vi "LibXML_ReadXMLTreeSerial.vi"(8 "error in":errorcluster, 9 "parent":u32, 10 "XML-tree in":T1[](array[typedef]), 11 "start node":u32) -> (0 "error out":errorcluster, 2 "XML-tree out":T1[](array[typedef]), 3 "copy of start node":u32)   [LabVIEW 2019, in "Tools.lvlib" / "LibXML.lvlib"]
uses:
  LibXML.lvlib
  LibXML_Element.ctl
  LibXML_Attribute.ctl
  LibXML_NavigateDirection.ctl
  LibXML_GetNodeStrPtr.vi
  LibXML_GetNodeResolvedContentStrPointer.vi
  LibXML_GetStringLength.vi
  LibXML_CopyString.vi
  Error Cluster From Error Code_subroutine.vi
  <vilib>/Utility/error.llb/Trim Whitespace.vi
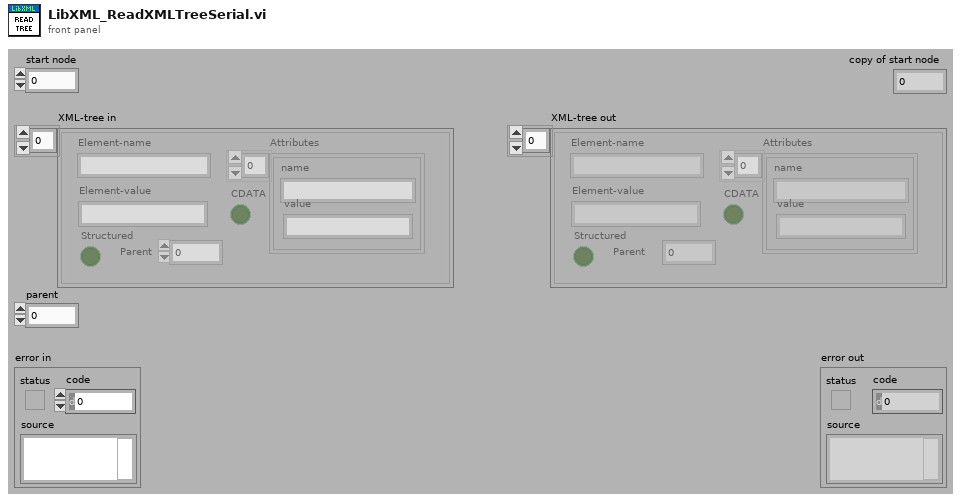
[diagram p1: front panel]
types:
  T1 = typedef "Tools.lvlib/LibXML.lvlib/LibXML_Element.ctl" = cluster{"Element-name":string, "Attributes":T2[], "Element-value":string, "CDATA":bool, "Parent":i32, "Structured":bool}
  T2 = typedef "Tools.lvlib/LibXML.lvlib/LibXML_Attribute.ctl" = cluster{"name":string, "value":string}
  T3 = typedef "Tools.lvlib/LibXML.lvlib/LibXML_NavigateDirection.ctl" = enum16{"NOP", "first child", "last child", "parent", "next", "prev"}
  T4 = enum16{"nothing", "element", "attribute", "text", "cdata", "5 or more"}
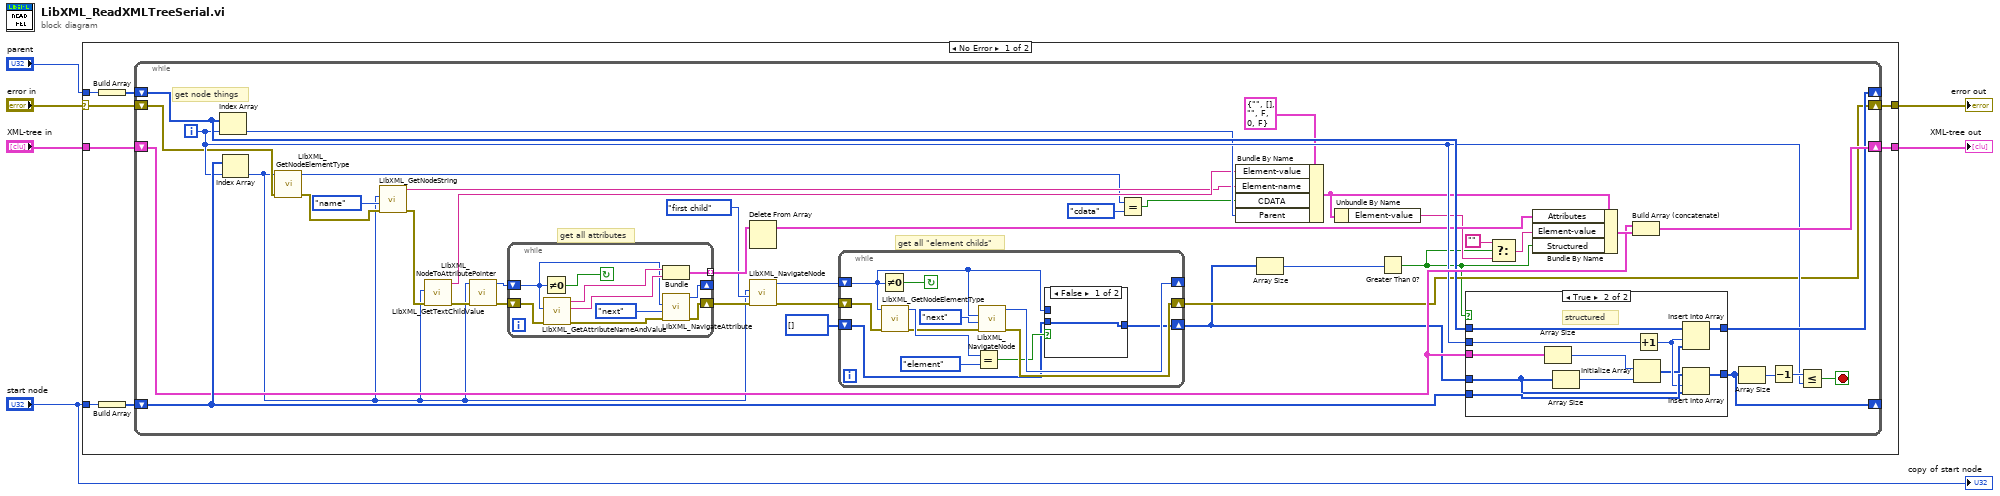
[diagram p0: block diagram]
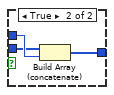
[diagram p2: hidden frame]
diagram:
  n1 = case shown="No Error" "error in" {
    selector: "error in" -> [w7 w96]
    tunnel: "XML-tree in" -> [w14 w95]
    tunnel: [w13 w95] -> w5
    tunnel: [w10 w96] -> w4
    tunnel: "parent" -> [w9 _]
    tunnel: "start node" -> [w8 _]
    frame No Error {
      n2 = Build Array(w9) -> (w11:u32[])
      n3 = Build Array(w8) -> (w12:u32[])
      n4 = while {
        shift-right: [w53] -> _
        shift-left: w12 -> [w52]
        shift-right: [w50] -> w13
        shift-left: w14 -> [w49]
        shift-right: [w48] -> _
        shift-left: w11 -> [w47]
        shift-right: [w24] -> w10
        shift-left: w7 -> [w37]
        i -> [w45]
        stop <- w55 stop-if-true
        # "get all \"element childs\""
        # "get all attributes"
        # "get node things"
        n5 = Index Array(array=w47, index=w45) -> (element=w31:u32)
        n6 = Index Array(array=w52, index=w45) -> (element=w16:u32)
        n7 = call "LibXML_GetNodeElementType.vi"("error in"=w37, "node"=w16) -> ("error out"=w36:errorcluster, "element type"=w15:T4)  [unwired: 7 in, 1 out]
        n8 = call "LibXML_GetNodeString.vi"("error in"=w36, "type"=enum16{"NOP", "name", "content"}."name", "node"=w16) -> ("error out"=w35:errorcluster, "lvstring"=w27:string)  [unwired: 7 in]
        n9 = call "LibXML_GetTextChildValue.vi"("error in"=w35, "node"=w16) -> ("error out"=w34:errorcluster, "lvstring"=w28:string)  [unwired: 4 in]
        n10 = call "LibXML_NodeToAttributePointer.vi"("error in"=w34, "node  in"=w16) -> ("error out"=w33:errorcluster, "attr out"=w42:u32)  [unwired: 8 in]
        n11 = while {
          shift-right: [w77] -> _
          shift-left: w42 -> [w73]
          tunnel: [w76] -> w41 mode=indexing
          shift-right: [w72] -> w25
          shift-left: w33 -> [w75]
          stop <- w81 continue-if-true
          n12 = Not Equal To 0?(x=w73) -> (x != 0?=w81:bool)
          n13 = call "LibXML_GetAttributeNameAndValue.vi"("error in"=w75, "attribute"=w73) -> ("error out"=w74:errorcluster, "value"=w79:string, "name"=w80:string)  [unwired: 7 in]
          n14 = Bundle("name"=w80, "value"=w79) -> (w76:cluster{"name":string, "value":string})  [unwired: 1 in]
          n15 = call "LibXML_NavigateAttribute.vi"("error in"=w74, "direction"=LibXML_NavigateDirection."next", "attribute in"=w73) -> ("error out"=w72:errorcluster, "attribute out"=w77:u32)  [unwired: 7 in]
        }
        n16 = Delete From Array(array=w41) -> (array with subset deleted=w40:cluster{"name":string, "value":string}[])  [unwired: 2 in, 1 out]
        n17 = call "LibXML_NavigateNode.vi"("error in (no error)"=w25, "direction"=LibXML_NavigateDirection."first child", "node in"=w16) -> ("error out"=w26:errorcluster, "node out"=w39:u32)  [unwired: 2 in, 1 out]
        n18 = while {
          shift-right: [w64] -> _
          shift-left: w39 -> [w58]
          shift-right: [w62] -> w24
          shift-left: w26 -> [w60]
          shift-right: [w57] -> w19
          shift-left: u32[] [] -> [w56]
          stop <- w63 continue-if-true
          n19 = Not Equal To 0?(x=w58) -> (x != 0?=w63:bool)
          n20 = call "LibXML_GetNodeElementType.vi"("error in"=w60, "node"=w58) -> ("error out"=w61:errorcluster, "element type"=w66:T4)  [unwired: 7 in, 1 out]
          n21 = Equal?(x=w66, y=T4."element") -> (x = y?=w59:bool)
          n22 = call "LibXML_NavigateNode.vi"("error in (no error)"=w61, "direction"=LibXML_NavigateDirection."next", "node in"=w58) -> ("error out"=w62:errorcluster, "node out"=w64:u32)  [unwired: 2 in, 1 out]
          n23 = case shown="False" w59 {
            tunnel: w58 -> [_ w71]
            tunnel: [w68 w70] -> w57
            tunnel: w56 -> [w68 w69]
            frame False {
            }
            frame True {
              n24 = Build Array (concatenate)(w69, w71) -> (w70:u32[])
            }
          }
        }
        n25 = Equal? ("Cdata?")(x=w15, y=T4."cdata") -> (x = y?=w30:bool)
        n26 = Bundle By Name(cluster=T1 {"Element-name"="", "Attributes"=[], "Element-value"="", "CDATA"=FALSE, "Parent"=0, "Structured"=FALSE} ("Element (for type)"), "Element-value"=w28, "Element-name"=w27, "CDATA"=w30, "Parent"=w31) -> (w29:T1)
        n27 = Array Size(array=w19) -> (size(s)=w18:i32)
        n28 = Unbundle By Name(w29) -> ("Element-value"=w22:string)
        n29 = Greater Than 0?(x=w18) -> (x > 0?=w17:bool)
        n30 = case shown="True" w17 {
          tunnel: w19 -> [_ w89]
          tunnel: [w83 w88] -> w53
          tunnel: w52 -> [w83 w90]
          tunnel: w45 -> [_ w94]
          tunnel: w49 -> [_ w93]
          tunnel: [w82 w84] -> w48
          tunnel: w47 -> [w82 w87]
          frame False {
            # "Not structured"
          }
          frame True {
            # "structured"
            n31 = Array Size(array=w93) -> (size(s)=w91:i32)
            n32 = Array Size(array=w89) -> (size(s)=w92:i32)
            n33 = Initialize Array(w91, w92) -> (w85:i32[])
            n34 = Increment(x=w94) -> (x+1=w86:i32)
            n35 = Insert Into Array(array=w87, index=w86, new element=w85) -> (w84:u32[])
            n36 = Insert Into Array(array=w90, index=w86, new element=w89) -> (w88:u32[])
          }
        }
        n37 = Select(t="", s=w17, f=w22) -> (s? t:f=w21:string)
        n38 = Bundle By Name(cluster=w29, "Attributes"=w40, "Element-value"=w21, "Structured"=w17) -> (w51:T1)
        n39 = Build Array (concatenate)(w49, w51) -> (w50:T1[])
        n40 = Array Size(array=w53) -> (size(s)=w54:i32)
        n41 = Decrement(x=w54) -> (x-1=w46:i32)
        n42 = Less Or Equal?(x=w46, y=w45) -> (x <= y?=w55:bool)
      }
    }
    frame Error {
    }
  }
  "error out" <- w4
  "XML-tree out" <- w5
  "copy of start node" <- "start node"
